vi "append_audio.vi"(4 "latest":waveform(dbl)[](array[waveform]), 5 "Old":waveform(dbl)[](array[waveform])) -> (1 "Appended":waveform(dbl)[](array[waveform]))   [LabVIEW 2020]
uses:
  <vilib>/Waveform/WDTOps.llb/WDT Append Waveforms DBL.vi
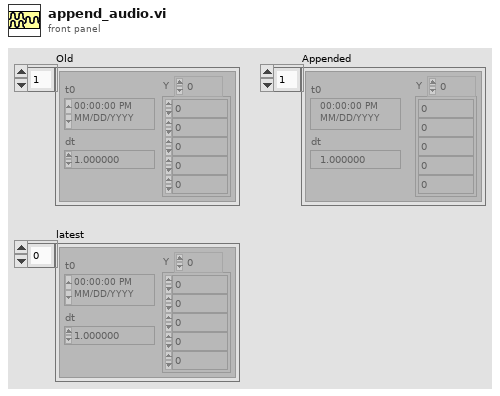
[diagram p1: front panel]
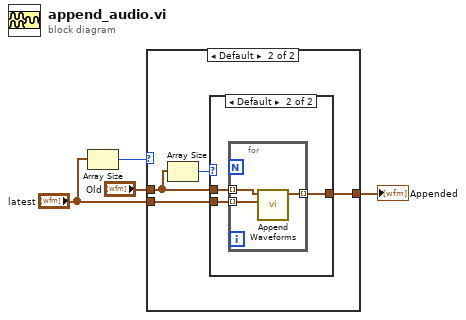
[diagram p0: block diagram]
diagram:
  n1 = Array Size(array="latest") -> (size(s)=w1:i32)
  n2 = case shown="Default" w1 {
    tunnel: [w5 w9] -> w4
    tunnel: "Old" -> [w5 w7]
    tunnel: "latest" -> [_ w8]
    frame 0 {
    }
    frame Default {
      n3 = Array Size(array=w7) -> (size(s)=w6:i32)
      n4 = case shown="Default" w6 {
        tunnel: [w10 w13] -> w9
        tunnel: w8 -> [w10 w12]
        tunnel: w7 -> [_ w11]
        frame 0 {
        }
        frame Default {
          n5 = for {
            tunnel: w11 -> [w16] mode=indexing
            tunnel: w12 -> [w15] mode=indexing
            tunnel: [w14] -> w13 mode=indexing
            n6 = call-poly <vilib>:"Append Waveforms.vi"("waveform B"=w15, "waveform A"=w16) -> ("waveform out"=w14:waveform(dbl))  [unwired: 8 in, 1 out]
          }
        }
      }
    }
  }
  "Appended" <- w4
